vi "Cluster_to_Strings.vi"(3 "Cluster":variant) -> (1 "Strings":string[][](array[string]))   [LabVIEW 2011, in "Third Party VIs.lvlib" / "pcardinale.lvlib"]
doc: "Takes any cluster, returns a 2-D array of strings:\nColumn 0 containing the names of the components (in hierarchal dot notation),\ncolumn 1 containing the names of the types,\nand column 2 containing the values."
uses:
  pcardinale.lvlib
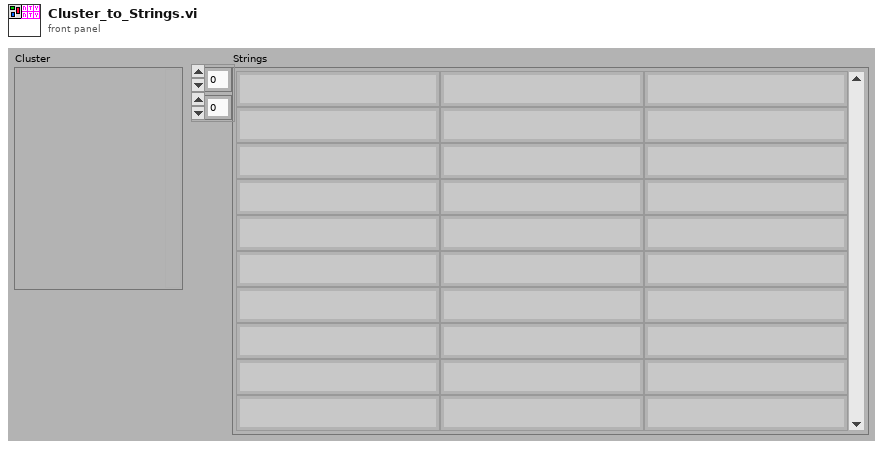
[diagram p1: front panel]
types:
  T1 = cluster{"status":bool, "code":i32, "source":string, "Inner":cluster{"floats":dbl[][], "file":path, "Other":cluster{"enum x":enum32{"x1", "x2"}, "cpx":cxt}}}
  T2 = typedef "Third Party VIs.lvlib/pcardinale.lvlib/XML_Item_Type.ctl" = enum16{"String", "Start Tag", "Stop Tag", "Unified Tag"}
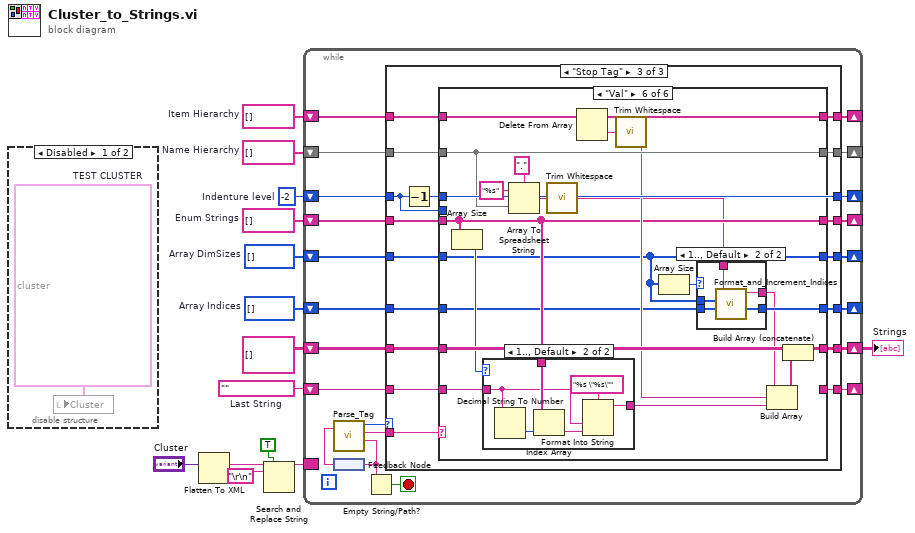
[diagram p0: block diagram]
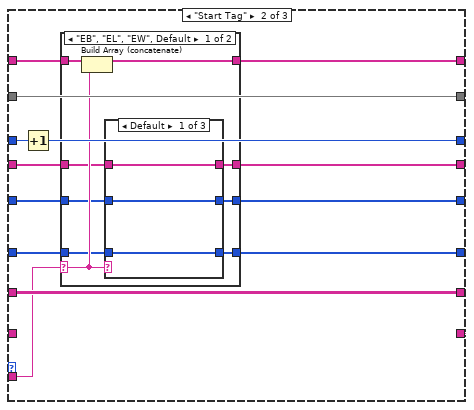
[diagram p3: hidden frame]
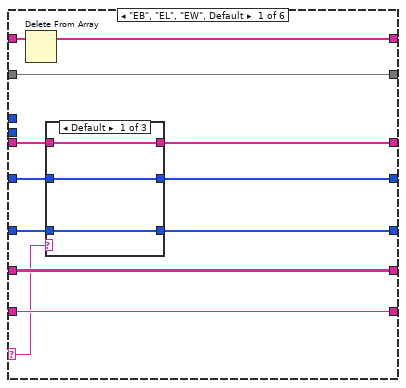
[diagram p7: hidden frame]
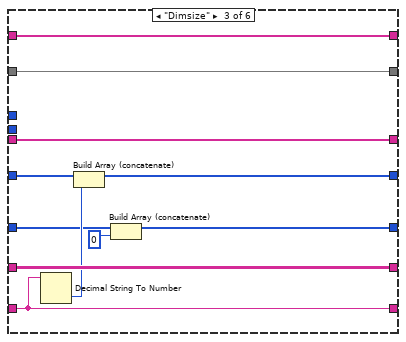
[diagram p11: hidden frame]
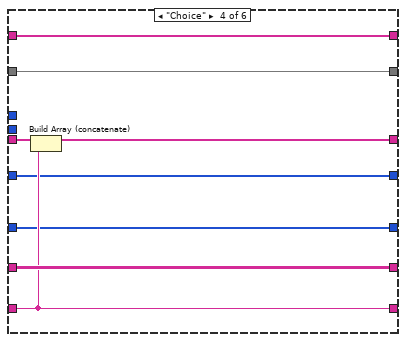
[diagram p12: hidden frame]
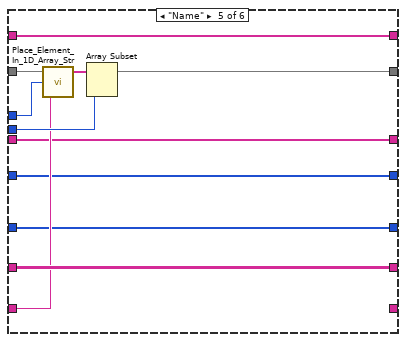
[diagram p13: hidden frame]
diagram:
  w1 = i32[] []  # Array Indices
  w2 = i32[] []  # Array DimSizes
  w3 = string[] []  # Enum Strings
  w4 = string[] []  # Item Hierarchy
  w5 = string[] []  # Name Hierarchy
  w6 = -2  # Indenture level
  w7 = ""  # Last String
  n1 = disable-structure shown="Disabled" {
    frame Disabled {
      w15 = T1 {"status"=TRUE, "code"=123, "source"="ABCDEF", "Inner"={"floats"=[[1.0, 2.0, 3.0], [0.0, 0.0, 5.0]], "file"=path "C:/temp", "Other"={"enum x"=enum."x2", "cpx"=12.0+34.0i}}}  # TEST CLUSTER
      n2 = local write "Cluster"(w15) -> ()
    }
    frame Enabled {
    }
  }
  n3 = Flatten To XML(anything="Cluster") -> (xml string=w8:string)
  n4 = Search and Replace String(replace all?=TRUE ("replace all? (F)"), input string=w8, search string="\r\n") -> (result string=w12:string)  [unwired: 5 in, 3 out]
  n5 = while {
    border: w12 -> [_]
    shift-right: [w31] -> w10
    shift-left: string[][] [] -> [w30]
    shift-right: [w28] -> _
    shift-left: w7 -> [w29]
    shift-right: [w26] -> _
    shift-left: w6 -> [w27]
    shift-right: [w24] -> _
    shift-left: w5 -> [w25]
    shift-right: [w22] -> _
    shift-left: w4 -> [w23]
    shift-right: [w20] -> _
    shift-left: w3 -> [w21]
    shift-right: [w18] -> _
    shift-left: w2 -> [w19]
    shift-right: [w16] -> _
    shift-left: w1 -> [w17]
    stop <- w35 stop-if-true
    n6 = feedback #1() -> (w36:string)
    n7 = call "Parse_Tag.vi"("String"=w36) -> ("Item Type"=w33:T2, "Item"=w32:string, "Remaining String"=w34:string)  [unwired: 2 in]
    n8 = feedback-in #1(w34) -> ()
    n9 = Empty String/Path?(string/path=w34) -> (empty?=w35:bool)
    n10 = case shown="\"Stop Tag\"" w33 {
      tunnel: w32 -> [w42 w45 w91]
      tunnel: [w44 w58 w93] -> w31
      tunnel: w30 -> [w44 w58 w94]
      tunnel: w29 -> [_ _ w92]
      tunnel: [w42 "" w90] -> w28
      tunnel: w27 -> [w43 w56 w84]
      tunnel: [w43 w52 w89] -> w26
      tunnel: w25 -> [w41 w55 w88]
      tunnel: [w41 w55 w87] -> w24
      tunnel: w23 -> [w40 w54 w86]
      tunnel: [w40 w53 w85] -> w22
      tunnel: w21 -> [w39 w51 w83]
      tunnel: [w39 w50 w82] -> w20
      tunnel: w19 -> [w38 w49 w81]
      tunnel: [w38 w48 w80] -> w18
      tunnel: w17 -> [w37 w47 w79]
      tunnel: [w37 w46 w78] -> w16
      frame Default {
      }
      frame "Start Tag" {
        n11 = Increment(x=w56) -> (x+1=w52:i32)
        n12 = case shown="\"EB\", \"EL\", \"EW\", Default" w45 {
          selector: w45 -> [w65 _]
          tunnel: w54 -> [w67 w77]
          tunnel: [w66 w77] -> w53
          tunnel: w51 -> [w64 w76]
          tunnel: [w63 w76] -> w50
          tunnel: w49 -> [w62 w75]
          tunnel: [w61 w75] -> w48
          tunnel: w47 -> [w60 w74]
          tunnel: [w59 w74] -> w46
          frame "EB", "EL", "EW", Default {
            n13 = Build Array (concatenate)(w67, w65) -> (w66:string[])
            n14 = case shown="Default" w65 {
              tunnel: w64 -> [w70 w71 _]
              tunnel: [w70 w71 _] -> w63
              tunnel: w62 -> [w69 _ w73]
              tunnel: [w69 _ w73] -> w61
              tunnel: w60 -> [w68 _ w72]
              tunnel: [w68 _ w72] -> w59
              frame Default {
              }
              frame "Array" {
              }
              frame "EB", "EL", "EW" {
              }
            }
          }
          frame "Choice", "Dimsize", "Name", "NumElts", "Val" {
          }
        }
      }
      frame "Stop Tag" {
        n15 = Decrement(x=w84) -> (x-1=w89:i32)
        n16 = case shown="\"Val\"" w91 {
          selector: w91 -> [w101 _ _ _ _ _]
          tunnel: w92 -> [w104 w115 w126 w135 w142 w157]
          tunnel: [w106 w119 w130 w138 w149 w168] -> w93
          tunnel: w94 -> [w106 w119 w130 w138 w149 w167]
          tunnel: [w104 w115 w126 w135 _ _] -> w90
          tunnel: w89 -> [_ _ _ _ w148 _]
          tunnel: w88 -> [w105 w118 w129 w137 w145 w164]
          tunnel: [w105 w118 w129 w137 w144 w164] -> w87
          tunnel: w86 -> [w103 w117 w128 w136 w146 w161]
          tunnel: [w102 w117 w128 w136 w146 w160] -> w85
          tunnel: w84 -> [_ _ _ _ w147 _]
          tunnel: w83 -> [w100 w116 w127 w134 w141 w158]
          tunnel: [w99 w116 w127 w133 w141 w158] -> w82
          tunnel: w81 -> [w98 w113 w125 w132 w140 w150]
          tunnel: [w97 w113 w123 w132 w140 w150] -> w80
          tunnel: w79 -> [w96 w114 w122 w131 w139 w155]
          tunnel: [w95 w114 w120 w131 w139 w154] -> w78
          frame "EB", "EL", "EW", Default {
            n17 = Delete From Array(array=w103) -> (array with subset deleted=w102:string[])  [unwired: 2 in, 1 out]
            n18 = case shown="Default" w101 {
              tunnel: w100 -> [w109 w110 _]
              tunnel: [w109 w110 _] -> w99
              tunnel: w98 -> [w108 _ w112]
              tunnel: [w108 _ w112] -> w97
              tunnel: w96 -> [w107 _ w111]
              tunnel: [w107 _ w111] -> w95
              frame Default {
              }
              frame "Array" {
              }
              frame "EB", "EL", "EW" {
              }
            }
          }
          frame "NumElts" {
          }
          frame "Dimsize" {
            n19 = Decimal String To Number(string=w126) -> (number=w124:i32)  [unwired: 2 in, 1 out]
            n20 = Build Array (concatenate)(w125, w124) -> (w123:i32[])
            n21 = Build Array (concatenate)(w122, 0) -> (w120:i32[])
          }
          frame "Choice" {
            n22 = Build Array (concatenate)(w134, w135) -> (w133:string[])
          }
          frame "Name" {
            n23 = call "Place_Element_In_1D_Array_Str.vi"("element"=w142, "index"=w148, "String array in"=w145) -> ("String output array"=w143:string[])
            n24 = Array Subset(array=w143, length=w147) -> (w144:string[])  [unwired: 1 in]
          }
          frame "Val" {
            n25 = Array Size(array=w158) -> (size(s)=w159:i32)
            n26 = case shown="1.., Default" w159 {
              tunnel: w157 -> [w178 w180]
              tunnel: w158 -> [_ w181]
              tunnel: [w178 w179] -> w153
              frame 0 {
              }
              frame 1.., Default {
                n27 = Decimal String To Number(string=w180) -> (number=w182:i32)  [unwired: 2 in, 1 out]
                n28 = Index Array(array=w181, index=w182) -> (element=w183:string)
                n29 = Format Into String(format string="%s \"%s\"", w180, w183) -> (resulting string=w179:string)  [unwired: 2 in, 1 out]
              }
            }
            n30 = Array To Spreadsheet String(delimiter (Tab)=".", array=w164, 3:"%s" ("format string")) -> (spreadsheet string=w166:string)
            n31 = call <vilib>:"Trim Whitespace.vi"("string"=w166) -> ("trimmed string"=w152:string)  [unwired: 1 in]
            n32 = Delete From Array(array=w161) -> (deleted portion=w163:string, array with subset deleted=w160:string[])  [unwired: 2 in]
            n33 = call <vilib>:"Trim Whitespace.vi"("string"=w163) -> ("trimmed string"=w162:string)  [unwired: 1 in]
            n34 = Array Size(array=w150) -> (size(s)=w156:i32)
            n35 = case shown="1.., Default" w156 {
              tunnel: w152 -> [w172 w177]
              tunnel: [w172 w176] -> w151
              tunnel: w150 -> [_ w173]
              tunnel: w155 -> [w171 w175]
              tunnel: [w171 w174] -> w154
              frame 0 {
              }
              frame 1.., Default {
                n36 = call "Format_and_Increment_Indices.vi"("Indices"=w175, "DimSizes"=w173, "initial string"=w177) -> ("New Indices"=w174:i32[], "string w/ indices"=w176:string)  [unwired: 2 in, 1 out]
              }
            }
            n37 = Build Array(w151, w162, w153) -> (w165:string[])
            n38 = Build Array (concatenate)(w167, w165) -> (w168:string[][])
          }
        }
      }
    }
  }
  "Strings" <- w10
